vi "RemFilter Unit Test.vi"(8 "error in (no error)":errorcluster, 10 "Filter Name":string, 11 "Main Display in":refnum<class "Main Display.lvclass">) -> (0 "error out":errorcluster, 2 "Filter Name Array":string[](array[string]), 3 "Main Display out":refnum<class "Main Display.lvclass">)   [LabVIEW 2016, in "Assert API Components.lvlib" / "Assert Display.lvlib" / "Main Display.lvlib" / "Main Display.lvclass"]
uses:
  Core/Main Display/Main Display/Main Display.lvclass
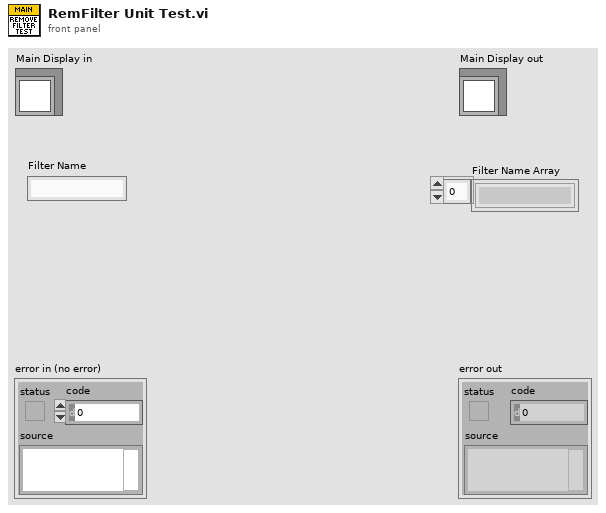
[diagram p1: front panel]
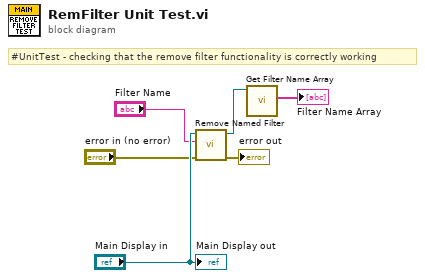
[diagram p0: block diagram]
diagram:
  # "#UnitTest - checking that the remove filter functionality is correctly working"
  n1 = call "Remove Named Filter.vi"("error in (no error)"="error in (no error)", "Filter Name"="Filter Name", "Main Display in"="Main Display in") -> ("error out"=→"error out":errorcluster, "Main Display out"=w6:refnum<class "Main Display.lvclass">)  [unwired: 7 in]
  n2 = call "Get Filter Name Array.vi"("Main Display in"=w6) -> ("Filter Name Array"=→"Filter Name Array":string[])  [unwired: 10 in]
  "Main Display out" <- "Main Display in"
